vi "Disable.vi"(8 "error in (no error)":errorcluster, 11 "NhRegenGridSim in":refnum<class "NHRGridSim.lvclass">) -> (0 "error out":errorcluster, 3 "NhRegenGridSim out":refnum<class "NHRGridSim.lvclass">)   [LabVIEW 2018, in "AcPwrPlugins.lvlib" / "NHRGridSim.lvclass"]
doc: "This VI turns off the unit. Off is defined as the output relay being open."
uses:
  NHRGridSim.lvclass
  <instrlib>/NH Research 9400 Series/NH Research 9400 Series.lvlib
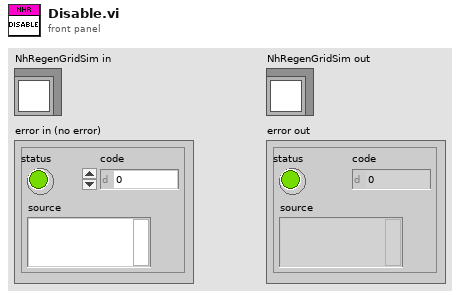
[diagram p1: front panel]
types:
  T1 = typedef "AcPwrPlugins.lvlib/NHRGridSim.lvclass/NHRGrid_Device(s)Settings.ctl" = cluster{"MeasName":string, "Hardware":T2}
  T2 = typedef "AcPwrPlugins.lvlib/NHRGridSim.lvclass/NHRGrid_Hardware.ctl" = cluster{"Handle":string, "Reset":bool, "Mode":T3, "ID Query":bool, "Connected":bool, "Logical Instrument":T4}
  T3 = typedef "AcPwrPlugins.lvlib/NHRGridSim.lvclass/NHRGrid_Modes.ctl" = u8
  T4 = typedef "AcPwrPlugins.lvlib/NHRGridSim.lvclass/NHRGrid_Logical_Instrument.ctl" = T5[]
  T5 = typedef "AcPwrPlugins.lvlib/NHRGridSim.lvclass/NHRGrid_InstrumentCluster.ctl" = cluster{"Name":string, "Vout (V)":dbl, "VType":string, "Phases":T6, "Slew Rates":T7, "FreqOut (Hz)":dbl, "Aperture (cycles)":i32, "Configure Instrument":enum32{"Conf1", "Conf2", "Conf3"}, "AC Wave Shape":enum32{"Sine", "User1", "User2", "User3"}, "Ranges":T8, "Safety Trips":T9, "Watchdog":T10}
  T6 = typedef "AcPwrPlugins.lvlib/NHRGridSim.lvclass/NHRGrid_Phases.ctl" = cluster{"A-Volts (V)":dbl, "B-Volts (V)":dbl, "C-Volts (V)":dbl, "Change at (Deg)":dbl, "B-Angle (Deg)":dbl, "C-Angle (Deg)":dbl}
  T7 = typedef "AcPwrPlugins.lvlib/NHRGridSim.lvclass/NHRGrid_SlewRates.ctl" = cluster{"Vmax (V/s)":dbl, "Vmin (V/s)":dbl, "Imax (A/s)":dbl, "Imin (A/s)":dbl, "Pmax (W/s)":dbl, "Pmin (W/s)":dbl, "Freq Max (Hz/s)":dbl, "Freq Min (Hz/s)":dbl, "Phase Angle Max (Deg/s)":dbl, "Phase Angle Min (Deg/s)":dbl}
  T8 = typedef "AcPwrPlugins.lvlib/NHRGridSim.lvclass/NHRGrid_Ranges.ctl" = cluster{"Voltage (V)":bool, "VHi":dbl, "Current (A)":bool, "CLo":dbl, "CHi":dbl, "VLo":dbl}
  T9 = typedef "AcPwrPlugins.lvlib/NHRGridSim.lvclass/NHRGrid_SafetyTrips.ctl" = cluster{"Vmax (V)":dbl, "Vmin (V)":dbl, "Vmax Time (s)":dbl, "Vmin Time (s)":dbl, "Imax Source (A)":dbl, "Imax Sink (A)":dbl, "Imax Source Time (s)":dbl, "Imax Sink Time (s)":dbl, "Pmax Source (W)":dbl, "Pmax Sink (W)":dbl, "Pmax Source Time (s)":dbl, "Pmax Sink Time (s)":dbl, "Absolute Volt Peak":dbl, "Enable Volt Peak":bool, "Absolute Curr Peak":dbl, "Enable Curr Peak":bool, "Setting t":string, "Recomm t 2":string}
  T10 = typedef "AcPwrPlugins.lvlib/NHRGridSim.lvclass/NHRGrid_Watchdog.ctl" = cluster{"Robust":bool, "Interval (s)":dbl}
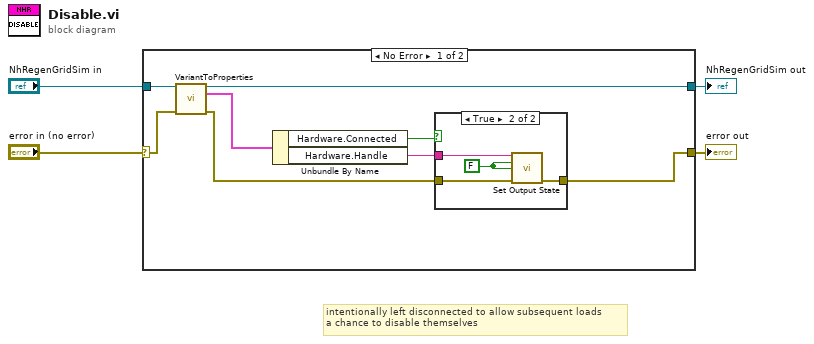
[diagram p0: block diagram]
diagram:
  # "intentionally left disconnected to allow subsequent loads\na chance to disable themselves"
  n1 = case shown="No Error" "error in (no error)" {
    selector: "error in (no error)" -> [w10 w19]
    tunnel: [w5 w19] -> w4
    tunnel: [w11 w18] -> w3
    tunnel: "NhRegenGridSim in" -> [w12 w18]
    frame No Error {
      n2 = call "VariantToProperties.vi"("NHRGridSim in"=w12, "error in (no error)"=w10) -> ("NHRGridSim out"=w11:refnum<class "NHRGridSim.lvclass">, "Device(s)Settings"=w8:T1, "error out"=w9:errorcluster)  [unwired: 8 in, 3 out]
      n3 = Unbundle By Name(w8) -> ("Hardware.Connected"=w6:bool, "Hardware.Handle"=w7:string)
      n4 = case shown="True" w6 {
        tunnel: w9 -> [w13 w14]
        tunnel: [w13 w17] -> w5
        tunnel: w7 -> [_ w15]
        frame False {
        }
        frame True {
          w16 = FALSE ("Output State (F: Disable)")
          n5 = call <instrlib>:"Set Output State.vi"("VISA resource name"=w15, "Output State (F: Disable)"=w16, "All (F: Disable)"=w16, "error in (no error)"=w14) -> ("error out"=w17:errorcluster)  [unwired: 10 in, 1 out]
        }
      }
    }
    frame Error {
    }
  }
  "error out" <- w4
  "NhRegenGridSim out" <- w3
